vi "WiiBalanceBoard_Calibration.vi"(0 "hWiimoteHandle in":u32 format="%08x", 1 "error in":errorcluster) -> (2 "hWiimoteHandle out":u32 format="%08x", 3 "Wii Balance Board Zeros":T1, 4 "error out":errorcluster)   [LabVIEW 2010]
doc: "CETPD\nThis VI read 100 samples of the sensors without nothing (zero weight) over the balance board, and computes the mean.\nX=0, Y=0 on the board"
uses:
  Wiimote Reporting Mode.ctl
  <vilib>/Analysis/NI_AALBase.lvlib
panel:
  out "output cluster":cluster{i16, i16, i16, i16}
  out "left-bottom zero":i16
  out "left-top zero":i16
  out "right-bottom zero":i16
  out "right-top zero":i16
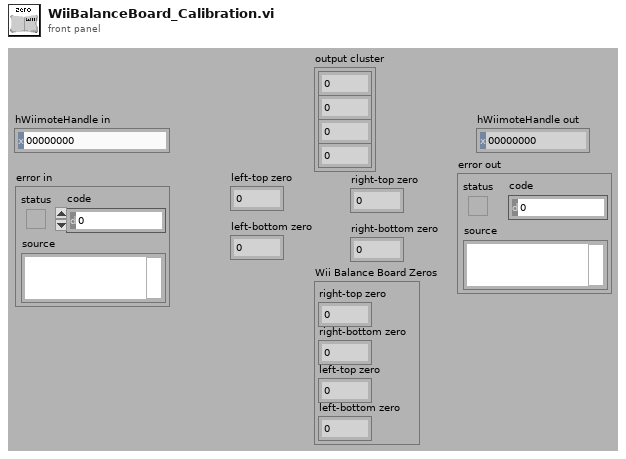
[diagram p1: front panel]
types:
  T1 = cluster{"right-top zero":i16, "right-bottom zero":i16, "left-top zero":i16, "left-bottom zero":i16}
  T2 = typedef "Wiimote Reporting Mode.ctl" = u8
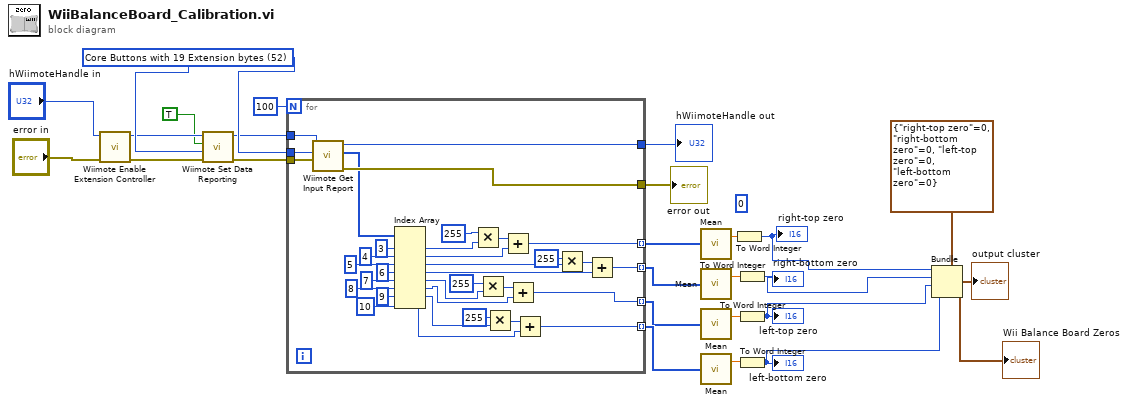
[diagram p0: block diagram]
diagram:
  (unwired) i16 0 ("unit (none)")
  w20 = T2 52 items=["Status Information"=32, "Read Data"=33, "Write Data"=34, "Core Buttons"=48, "Core Buttons and Accelerometer"=49, "Core Buttons with 8 Extension bytes"=50, "Core Buttons and Accelerometer with 12 IR bytes"=51, "Core Buttons with 19 Extension bytes"=52, "Core Buttons and Accelerometer with 16 Extension Bytes"=53, "Core Buttons with 10 IR bytes and 9 Extension Bytes"=54, "Core Buttons and Accelerometer with 10 IR bytes and 6 Extension Bytes"=55] ("Reporting Mode")
  n1 = call "Wiimote Enable Extension Controller.vi"("error in"="error in", "hWiimoteHandle in"="hWiimoteHandle in") -> ("error out"=w13:errorcluster, "hWiimoteHandle out"=w12:u32)  [unwired: 8 in]
  n2 = call "Wiimote Set Data Reporting.vi"("error in"=w13, "Reporting Mode"=w20, "Continuous"=TRUE, "hWiimoteHandle in"=w12) -> ("error out"=w17:errorcluster, "hWiimoteHandle out"=w16:u32)  [unwired: 6 in]
  n3 = for {
    N: 100 -> [_]
    tunnel: w16 -> [w59]
    tunnel: w17 -> [w58]
    tunnel: [w57] -> w18
    tunnel: [w56] -> w19
    tunnel: w20 -> [w55]
    tunnel: [w30] -> w21 mode=indexing
    tunnel: [w28] -> w22 mode=indexing
    tunnel: [w27] -> w23 mode=indexing
    tunnel: [w26] -> w24 mode=indexing
    n4 = call "Wiimote Get Input Report.vi"("error in"=w58, "bInputReport"=w55, "hWiimoteHandle in"=w59) -> ("error out"=w56:errorcluster, "pReportBuffer out"=w29:u8[], "hWiimoteHandle out"=w57:u32)  [unwired: 6 in]
    n5 = Index Array(array=w29, index #1=3 ("index"), index #2=4 ("index"), index #3=5 ("index"), index #4=6 ("index"), index #5=7 ("index"), index #6=8 ("index"), index #7=9 ("index"), index #8=10 ("index")) -> (element #1=w41:u8, element #2=w45:u8, element #3=w40:u8, element #4=w43:u8, element #5=w36:u8, element #6=w37:u8, element #7=w32:u8, element #8=w31:u8)
    n6 = Multiply(x=u16 255 ("y"), y=w41) -> (x*y=w46:u16)
    n7 = Multiply(x=u16 255 ("y"), y=w36) -> (x*y=w38:u16)
    n8 = Multiply(x=u32 255 ("y"), y=w32) -> (x*y=w34:u32)
    n9 = Add(x=w46, y=w45) -> (x+y=w30:u16)
    n10 = Add(x=w38, y=w37) -> (x+y=w27:u16)
    n11 = Add(x=w34, y=w31) -> (x+y=w26:u32)
    n12 = Multiply(x=u16 255 ("y"), y=w40) -> (x*y=w44:u16)
    n13 = Add(x=w44, y=w43) -> (x+y=w28:u16)
  }
  "hWiimoteHandle out" <- w18
  "error out" <- w19
  n14 = call <vilib>:"Mean.vi"("X"=w21) -> ("mean"=w7:dbl)  [unwired: 1 out]
  n15 = call <vilib>:"Mean.vi"("X"=w22) -> ("mean"=w10:dbl)  [unwired: 1 out]
  n16 = call <vilib>:"Mean.vi"("X"=w23) -> ("mean"=w9:dbl)  [unwired: 1 out]
  n17 = call <vilib>:"Mean.vi"("X"=w24) -> ("mean"=w8:dbl)  [unwired: 1 out]
  n18 = To Word Integer(number=w7) -> (16bit integer=w6:i16)
  "right-top zero" <- w6
  n19 = To Word Integer(number=w10) -> (16bit integer=w5:i16)
  "right-bottom zero" <- w5
  n20 = To Word Integer(number=w9) -> (16bit integer=w4:i16)
  "left-top zero" <- w4
  n21 = To Word Integer(number=w8) -> (16bit integer=w3:i16)
  "left-bottom zero" <- w3
  n22 = Bundle(cluster=T1 {"right-top zero"=0, "right-bottom zero"=0, "left-top zero"=0, "left-bottom zero"=0} ("Cluster"), "right-top zero"=w6, "right-bottom zero"=w5, "left-top zero"=w4, "left-bottom zero"=w3) -> (→"output cluster" →"Wii Balance Board Zeros":T1)
